vi "myRIO_BRig_RT_TCP__v2__noAnalog.vi"(0 "input_hTCP":refnum<k5>, 1 "input_AI1":i16, 2 "input_AI0":i16, 3 "input_I_connected_TCP":bool, 5 "input_iBlock":u16, 7 "input_spout":enum16{"Left", "Right"}(ring), 9 "input_iTrial":u16, 11 "input_error":errorcluster, 13 "input_iState":T1) -> (4 "output_hTCP":refnum<k5>, 15 "output_error":errorcluster)   [LabVIEW 2014]
uses:
  myRIO_BRig_RT__Case_Exp_stateList.ctl
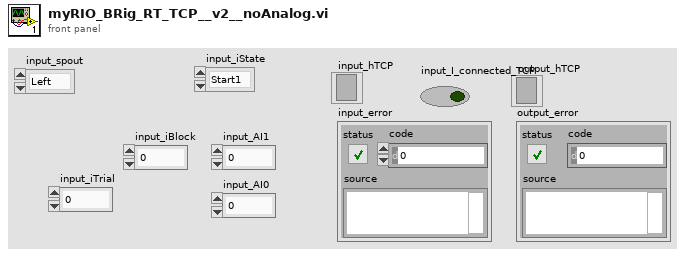
[diagram p1: front panel]
types:
  T1 = typedef "myRIO_BRig_RT__Case_Exp_stateList.ctl" = enum16{"Start1", "Start2", "Start3", "saveSettings1", "saveSettings2", "saveSettings3", "saveSettings4_LC_ENL", "saveSettings5_LC_Cue", "saveSettings6_LC_Other", "setSettings_Audio", "setSettings_Laser", "initBlock_pre", "initBlock", "initBlock2", "initBlock_post", "initTrial_pre", "initTrial", "initTrial2", "initTrial3", "initTrial4", "initTrial_LC_ENL1", "initTrial_LC_Cue1", "initTrial_LC_Sel", "initTrial_post", "ENL1_pre", "ENL1", "ENL1_post", "ENL1Penalty_pre", "ENL1Penalty", "ENL2_pre", "ENL2", "ENL2Penalty_pre", "ENL2Penalty", "Cue1_pre", "Cue1", "Cue1_post", "Cue1Penalty_pre", "Cue1Penalty", "Cue2_pre", "Cue2", "Cue2Penalty_pre", "Cue2Penalty", "Selection_pre", "Selection", "Select_post", "SelectReward_pre", "SelectReward", "SelectRewardPost_pre", "SelectRewardPost", "SelectWrong_pre", "SelectWrong", "SelectWrong_post", "SelectTimeout_pre", "SelectTimeout", "SelectTimeout_post", "endTrial_pre", "endTrial1", "endTrial2", "endTrial3", "endTrial_post", "endBlock_pre", "endBlock", "endBlock_post", "endExp", "commConnect", "commUpload_pre", "commUpload_dataBlock", "commUpload_dataCurrent", "commUpload_dataExp", "commUpload_dataLC", "commUpload_dataTrial", "commUpload_post", "saveData_pre", "saveData_dataBlock", "saveData_dataCurrent", "saveData_dataExp", "saveData_dataLC", "saveData_dataTrial", "saveData_post", "empty_endBlock1", "empty_endBlock2", "empty_endTrial1", "empty_endTrial2", "empty_endTrial3", "empty_endTrial4", "empty_endTrial5"}
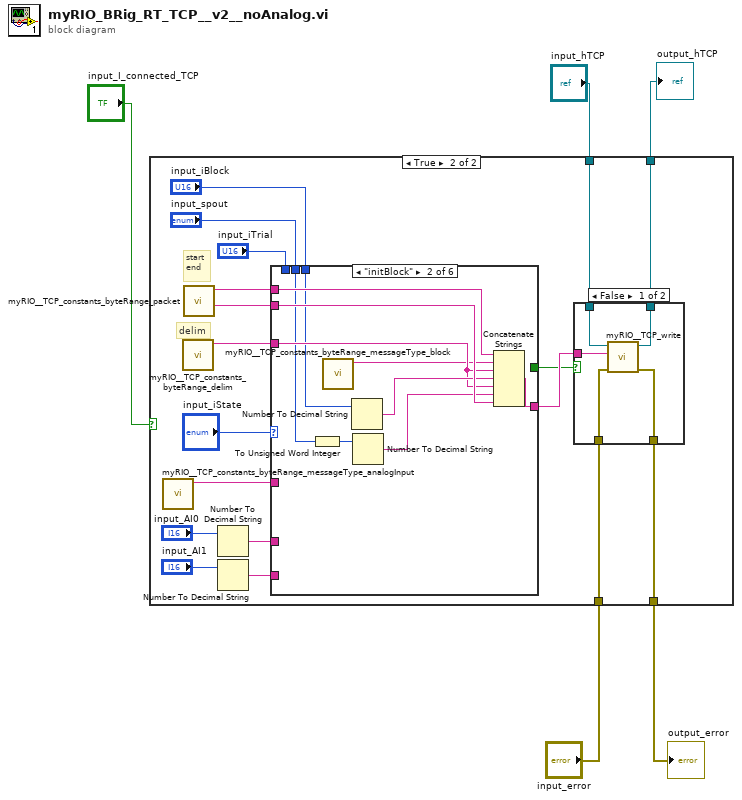
[diagram p0: block diagram]
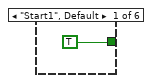
[diagram p4: hidden frame]
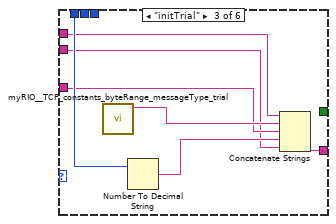
[diagram p5: hidden frame]
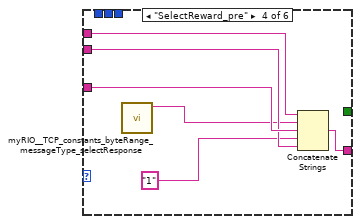
[diagram p6: hidden frame]
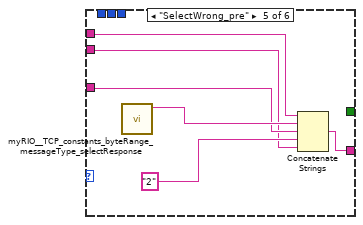
[diagram p7: hidden frame]
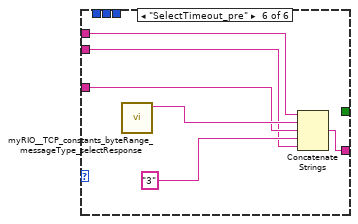
[diagram p8: hidden frame]
diagram:
  n1 = case shown="True" "input_I_connected_TCP" {
    tunnel: "input_hTCP" -> [w7 w25]
    tunnel: "input_error" -> [w6 w24]
    tunnel: [w7 w23] -> w3
    tunnel: [w6 w22] -> w2
    frame False {
    }
    frame True {
      # "start\nend"
      # "delim"
      n2 = call "myRIO__TCP_constants_byteRange_messageType_analogInput.vi"() -> ("output_analogInput_char"=w12:string)  [unwired: 10 in, 1 out]
      n3 = call "myRIO__TCP_constants_byteRange_delim.vi"() -> ("output_delim_char"=w18:string)  [unwired: 10 in, 1 out]
      n4 = call "myRIO__TCP_constants_byteRange_packet.vi"() -> ("output_end_char"=w19:string, "output_start_char"=w20:string)  [unwired: 8 in, 2 out]
      n5 = Number To Decimal String(number="input_AI0") -> (decimal integer string=w14:string)  [unwired: 1 in]
      n6 = Number To Decimal String(number="input_AI1") -> (decimal integer string=w13:string)  [unwired: 1 in]
      n7 = case shown="\"initBlock\"" "input_iState" {
        tunnel: w20 -> [_ w41 w48 w53 w57 w64]
        tunnel: w19 -> [_ w40 w44 w54 w58 w63]
        tunnel: w18 -> [_ w38 w46 w55 w59 w65]
        tunnel: [_ w42 w50 w56 w60 w66] -> w17
        tunnel: w14 -> [_ _ _ _ _ _]
        tunnel: w13 -> [_ _ _ _ _ _]
        tunnel: w12 -> [_ _ _ _ _ _]
        tunnel: "input_iTrial" -> [_ _ w49 _ _ _]
        tunnel: "input_spout" -> [_ w35 _ _ _ _]
        tunnel: "input_iBlock" -> [_ w36 _ _ _ _]
        tunnel: [TRUE _ _ _ _ _] -> w8
        frame "Start1", Default {
        }
        frame "initBlock" {
          n8 = To Unsigned Word Integer(number=w35) -> (unsigned 16bit integer=w43:u16)
          n9 = call "myRIO__TCP_constants_byteRange_messageType_block.vi"() -> ("output_Block_char"=w34:string)  [unwired: 10 in, 1 out]
          n10 = Number To Decimal String(number=w36) -> (decimal integer string=w39:string)  [unwired: 1 in]
          n11 = Number To Decimal String(number=w43) -> (decimal integer string=w37:string)  [unwired: 1 in]
          n12 = Concatenate Strings(w41, w34, w38, w39, w38, w37, w40) -> (w42:string)
        }
        frame "initTrial" {
          n13 = call "myRIO__TCP_constants_byteRange_messageType_trial.vi"() -> ("output_Trial_char"=w47:string)  [unwired: 10 in, 1 out]
          n14 = Number To Decimal String(number=w49) -> (decimal integer string=w45:string)  [unwired: 1 in]
          n15 = Concatenate Strings(w48, w47, w46, w45, w44) -> (w50:string)
        }
        frame "SelectReward_pre" {
          n16 = call "myRIO__TCP_constants_byteRange_messageType_selectResponse.vi"() -> ("output_selectResponse_char"=w51:string)  [unwired: 10 in, 1 out]
          n17 = Concatenate Strings(w53, w51, w55, "1", w54) -> (w56:string)
        }
        frame "SelectWrong_pre" {
          n18 = call "myRIO__TCP_constants_byteRange_messageType_selectResponse.vi"() -> ("output_selectResponse_char"=w61:string)  [unwired: 10 in, 1 out]
          n19 = Concatenate Strings(w57, w61, w59, "2", w58) -> (w60:string)
        }
        frame "SelectTimeout_pre" {
          n20 = call "myRIO__TCP_constants_byteRange_messageType_selectResponse.vi"() -> ("output_selectResponse_char"=w67:string)  [unwired: 10 in, 1 out]
          n21 = Concatenate Strings(w64, w67, w65, "3", w63) -> (w66:string)
        }
      }
      n22 = case shown="False" w8 {
        tunnel: w25 -> [w30 w32]
        tunnel: w24 -> [w29 w31]
        tunnel: [w28 w32] -> w23
        tunnel: [w27 w31] -> w22
        tunnel: w17 -> [w26 _]
        frame False {
          n23 = call "myRIO__TCP_write.vi"("input_error"=w29, "input_packet"=w26, "input_hTCP"=w30) -> ("output_error"=w27:errorcluster, "output_hTCP"=w28:refnum<k5>)  [unwired: 6 in, 1 out]
        }
        frame True {
        }
      }
    }
  }
  "output_hTCP" <- w3
  "output_error" <- w2
